vi "INI 2 Globals.vi"(11 "configuration file path":path) -> (0 "error out":errorcluster)   [LabVIEW 2014]
uses:
  <vilib>/Utility/config.llb/Read Key (String).vi
  <vilib>/Utility/config.llb/NI_LVConfig.lvlib
panel:
  out "IgnoreErrors":errorcluster
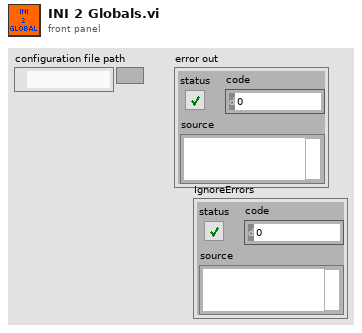
[diagram p1: front panel]
types:
  T1 = typedef "NI_LVConfig.lvlib/Config Data RefNum.ctl" = refnum<k1>
  T2 = enum32{"invalid VI type", "Standard VI", "Control VI", "Global VI", "Polymorphic VI", "Configuration VI", "SubSystem", "Facade VI", "Method VI", "Statechart Diagram VI"}
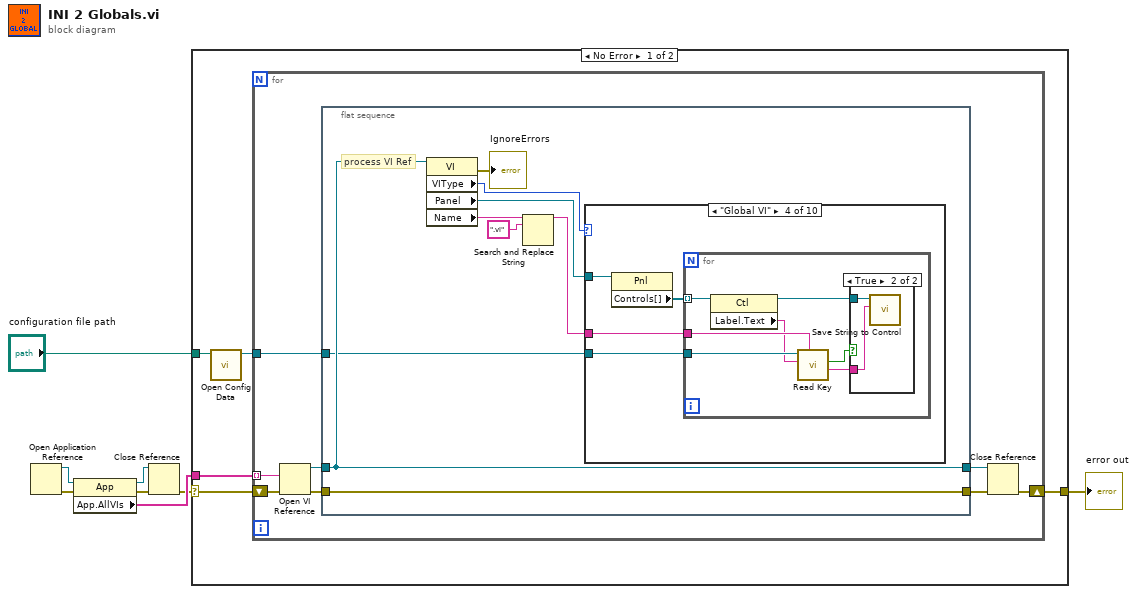
[diagram p0: block diagram]
diagram:
  n1 = Open Application Reference() -> (0:w4:errorcluster, 3:w1:refnum<vi>)  [unwired: 4 in]
  n2 = property class="App"(reference=w1, error in=w4) -> (reference out=w2:refnum<vi>, error out=w3:errorcluster, "App.AllVIs"=w6:string[])
  n3 = Close Reference(reference=w2, error in (no error)=w3) -> (error out=w5:errorcluster)
  n4 = case shown="No Error" w5 {
    selector: w5 -> [w12 w44]
    tunnel: w6 -> [w13 _]
    tunnel: [w11 w44] -> w7
    tunnel: "configuration file path" -> [w9 _]
    frame No Error {
      n5 = call <vilib>:"Open Config Data.vi"("configuration file path"=w9) -> ("refnum"=w10:T1)  [unwired: 8 in, 2 out]
      n6 = for {
        tunnel: w13 -> [w21] mode=indexing
        shift-right: [w15] -> w11
        shift-left: w12 -> [w16]
        tunnel: w10 -> [w14]
        n7 = Open VI Reference(vi path=w21, error in (no error)=w16) -> (vi reference=w20:refnum<vi>, error out=w18:errorcluster)  [unwired: 4 in]
        n8 = flat-sequence {
          tunnel: w20 -> [w29]
          tunnel: [w29] -> w19
          tunnel: w18 -> [w30]
          tunnel: [w30] -> w17
          tunnel: w14 -> [w23]
          frame #0 {
            # "process VI Ref"
            n9 = property class="VI"(reference=w29) -> (error out=→"IgnoreErrors":errorcluster, "VIType"=w28:T2, "Panel"=w27:refnum<vi>, "Name"=w26:string)  [unwired: 1 in, 1 out]
            n10 = Search and Replace String(input string=w26, search string=".vi" ("substring (\"\")")) -> (result string=w24:string)  [unwired: 6 in, 3 out]
            n11 = case shown="\"Global VI\"" w28 {
              tunnel: w27 -> [_ _ _ w34 _ _ _ _ _ _]
              tunnel: w24 -> [_ _ _ w31 _ _ _ _ _ _]
              tunnel: w23 -> [_ _ _ w32 _ _ _ _ _ _]
              frame "invalid VI type", Default {
              }
              frame "Standard VI" {
              }
              frame "Control VI" {
              }
              frame "Global VI" {
                n12 = property class="Pnl"(reference=w34) -> ("Controls[]"=w33:refnum<vi>[])  [unwired: 1 in, 2 out]
                n13 = for {
                  tunnel: w33 -> [w41] mode=indexing
                  tunnel: w32 -> [w39]
                  tunnel: w31 -> [w38]
                  n14 = property class="Ctl"(reference=w41) -> (reference out=w40:refnum<vi>, "Label.Text"=w37:string)  [unwired: 1 in, 1 out]
                  n15 = call-poly <vilib>:"Read Key.vi"("section"=w38, "key"=w37, "refnum"=w39) -> ("value"=w36:string, "found?"=w35:bool)  [unwired: 5 in, 2 out]
                  n16 = case shown="True" w35 {
                    tunnel: w40 -> [_ w43]
                    tunnel: w36 -> [_ w42]
                    frame False {
                    }
                    frame True {
                      n17 = call "Save String to Control.vi"("value"=w42, "Control"=w43) -> ()  [unwired: 10 in]
                    }
                  }
                }
              }
              frame "Polymorphic VI" {
              }
              frame "Configuration VI" {
              }
              frame "SubSystem" {
              }
              frame "Facade VI" {
              }
              frame "Method VI" {
              }
              frame "Statechart Diagram VI" {
              }
            }
          }
        }
        n18 = Close Reference(reference=w19, error in (no error)=w17) -> (error out=w15:errorcluster)
      }
    }
    frame Error {
    }
  }
  "error out" <- w7
